vi "Save File Extract Gain and Offset.vi"(11 "Analog Input":string) -> (3 "No Gain or Offset":string, 5 "Gain & Offset":string)   [LabVIEW 2016, in "File Setup.lvlib"]
uses:
  File Setup.lvlib
  <vilib>/Utility/error.llb/whitespace.ctl
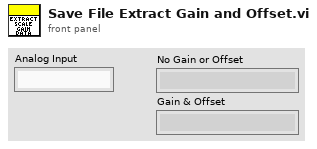
[diagram p1: front panel]
types:
  T1 = typedef "whitespace.ctl" = u16
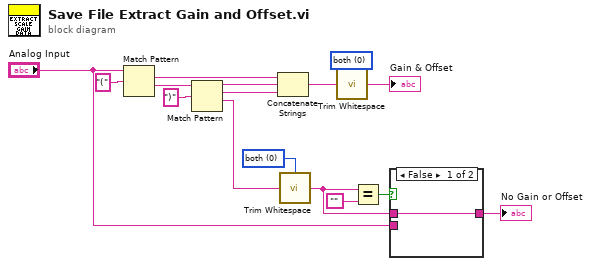
[diagram p0: block diagram]
diagram:
  w5 = T1 0 items=["both", "start of string", "end of string"] ("location (both)")
  w9 = T1 0 items=["both", "start of string", "end of string"] ("location (both)")
  n1 = Match Pattern(string="Analog Input", regular expression="(") -> (match substring=w14:string, after substring=w13:string)  [unwired: 1 in, 2 out]
  n2 = Match Pattern(string=w13, regular expression=")") -> (before substring=w15:string, match substring=w16:string, after substring=w4:string)  [unwired: 1 in, 1 out]
  n3 = Concatenate Strings(w14, w15, w16) -> (w10:string)
  n4 = call <vilib>:"Trim Whitespace.vi"("string"=w4, "location (both)"=w5) -> ("trimmed string"=w2:string)
  n5 = call <vilib>:"Trim Whitespace.vi"("string"=w10, "location (both)"=w9) -> ("trimmed string"=→"Gain & Offset":string)
  n6 = Equal?(x=w2, y="") -> (x = y?=w8:bool)
  n7 = case shown="False" w8 {
    tunnel: "Analog Input" -> [_ w18]
    tunnel: [w17 w18] -> w1
    tunnel: w2 -> [w17 _]
    frame False {
    }
    frame True {
    }
  }
  "No Gain or Offset" <- w1
